vi "GUILib.get library version.vi"() -> (0 "nameAndVersion":string)   [LabVIEW 2012, in "GUILib.lvlib"]
doc: "obtain name and version of a library as a string"
uses:
  GUILib.lvlib
  UtilityLib/UtilityLib.lvlib
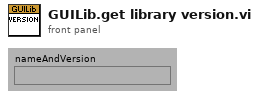
[diagram p1: front panel]
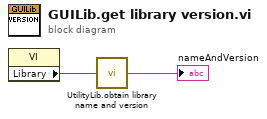
[diagram p0: block diagram]
diagram:
  n1 = property class="VI"() -> ("Library"=w1:refnum<vi>)  [unwired: 2 in, 2 out]
  n2 = call "UtilityLib.obtain library name and version.vi"("Library"=w1) -> ("nameAndVersion"=→"nameAndVersion":string)
